vi "Read SPI Digital Lines.vi"(0 "Chip Select DIO Lines":T1={"SCLK"="Port0/DIO3", "MISO"="Port0/DIO3", "MOSI"="Port0/DIO3", "CS 0"="Port0/DIO4", "CS 1"="Port0/DIO4", "CS 2"="Port0/DIO1", "CS 3"="Port0/DIO4", "CS 4"="Port0/DIO4", "CS 5"="Port0/DIO4"}, 11 "error in":errorcluster) -> (4 "Chip Select DIO Lines Out":T1={"SCLK"="Port0/DIO3", "MISO"="Port0/DIO3", "MOSI"="Port0/DIO3", "CS 0"="Port0/DIO4", "CS 1"="Port0/DIO4", "CS 2"="Port0/DIO1", "CS 3"="Port0/DIO4", "CS 4"="Port0/DIO4", "CS 5"="Port0/DIO4"}, 6 "SPI Read Data":T2, 15 "error out":errorcluster)   [LabVIEW 2014]
uses:
  <vilib>/eio/EIONode/EIONode.xnode
  <userlib>/_NI SPI IP/FPGA/Controllers/Public/Spi Master Inputs.ctl
  <userlib>/_NI SPI IP/FPGA/Controllers/NI SPI IP FPGA.lvlib
  <vilib>/rvi/eio/common/nirviEmuTemplateMethod_errors.vi
  SPI Digital IO Lines.ctl
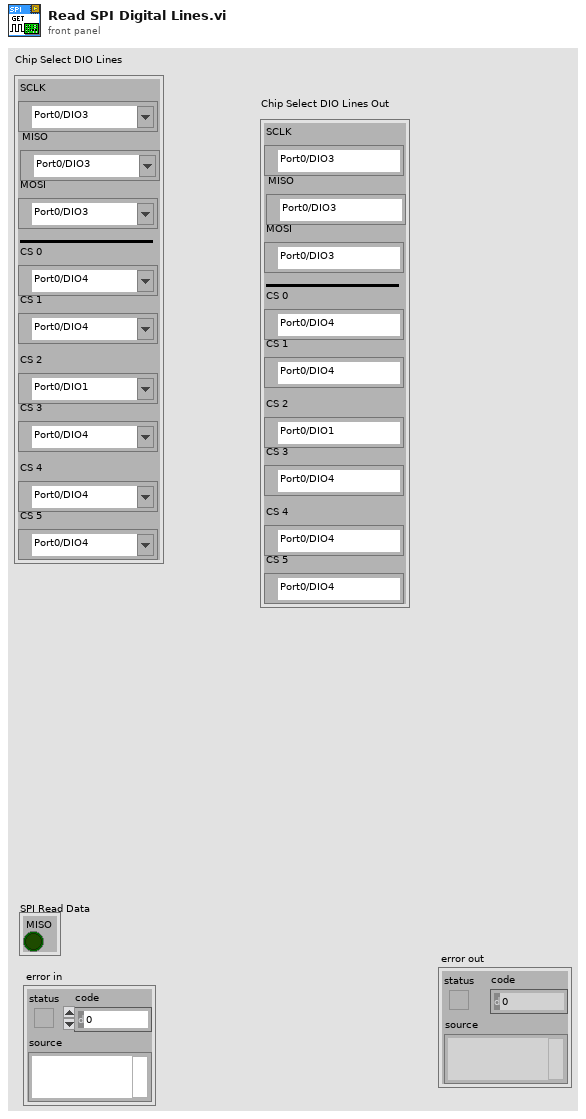
[diagram p1: front panel]
types:
  T1 = typedef "SPI Digital IO Lines.ctl" = cluster{"SCLK":refnum<k21>, "MISO":refnum<k21>, "MOSI":refnum<k21>, "CS 0":refnum<k21>, "CS 1":refnum<k21>, "CS 2":refnum<k21>, "CS 3":refnum<k21>, "CS 4":refnum<k21>, "CS 5":refnum<k21>}
  T2 = typedef "NI SPI IP FPGA.lvlib/Spi Master Inputs.ctl" = cluster{"MISO":bool}
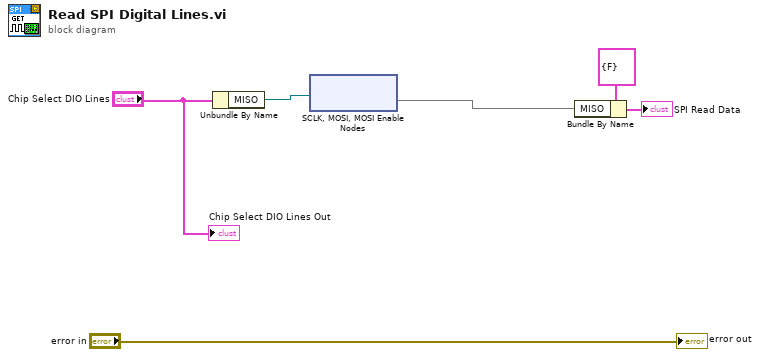
[diagram p0: block diagram]
diagram:
  n1 = Unbundle By Name("Chip Select DIO Lines") -> ("MISO"=w5:refnum<k21>)
  n2 = xnode "SCLK, MOSI, MOSI Enable Nodes"("FPGA I/O In"=w5) -> ("I/O Item"=w3)  [unwired: 1 out]
  n3 = Bundle By Name(cluster=T2 {"MISO"=FALSE} ("spi input"), "MISO"=w3) -> (→"SPI Read Data":T2)
  "Chip Select DIO Lines Out" <- "Chip Select DIO Lines"
  "error out" <- "error in"
